vi "Zero.vi"(0 "PM NI568X in":refnum<class "Power Meter.lvclass">, 11 "error in (no error)":errorcluster) -> (4 "PM NI568X out":refnum<class "Power Meter.lvclass">, 15 "error out":errorcluster)   [LabVIEW 2023, in "NI-568x RF Power Meter.lvlib" / "Power Meter.lvclass"]
uses:
  Power Meter.lvclass
  Power Meter.lvclass/Power Meter.ctl
  Properties/Read Resource Name.vi
  <vilib>/Utility/error.llb/Error Cluster From Error Code.vi
  <vilib>/ErrorRing/Error Ring.xnode
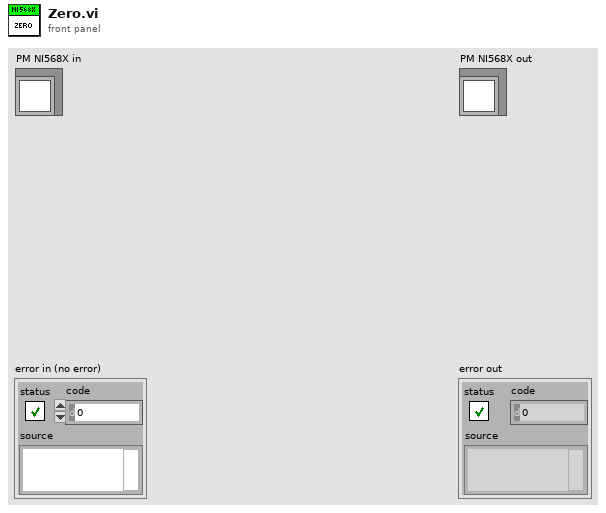
[diagram p1: front panel]
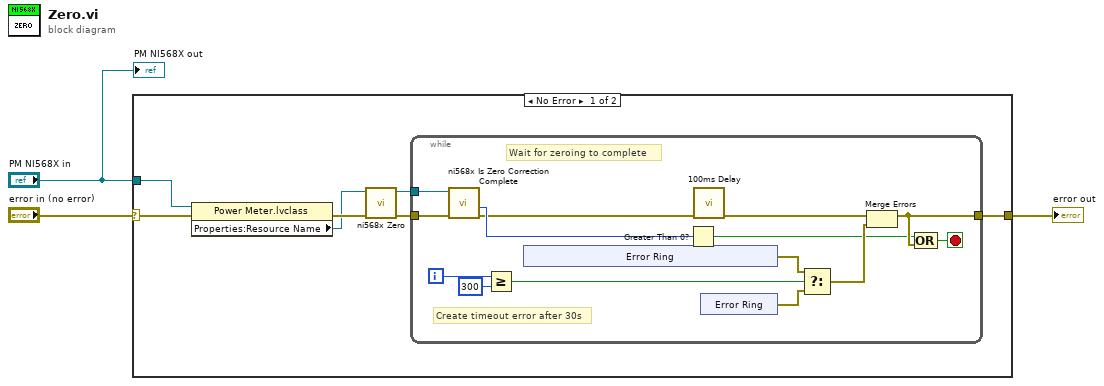
[diagram p0: block diagram]
diagram:
  n1 = case shown="No Error" "error in (no error)" {
    selector: "error in (no error)" -> [w7 w31]
    tunnel: [w8 w31] -> w3
    tunnel: "PM NI568X in" -> [w6 _]
    frame No Error {
      n2 = property class="Power Meter.lvclass"(reference=w6, error in=w7) -> (error out=w5:errorcluster, "Properties:Resource Name"=w4:refnum<k15>)  [unwired: 1 out]
      n3 = call <instrlib>:"ni568x Zero.vi"("error in"=w5, "instrument handle"=w4) -> ("error out"=w9:errorcluster, "instrument handle out"=w10:refnum<k15>)  [unwired: 8 in]
      n4 = while {
        tunnel: w9 -> [w24]
        tunnel: [w12] -> w8
        tunnel: w10 -> [w23]
        i -> [w22]
        stop <- w19 stop-if-true
        # "Create timeout error after 30s"
        # "Wait for zeroing to complete"
        n5 = call <instrlib>:"ni568x Is Zero Correction Complete.vi"("error in"=w24, "instrument handle"=w23) -> ("error out"=w18:errorcluster, "zero status"=w20:i32)  [unwired: 7 in, 1 out]
        n6 = Greater Or Equal?(x=w22, y=300) -> (x >= y?=w15:bool)
        n7 = xnode "Error Ring"() -> ("error out"=w16:errorcluster)
        n8 = Greater Than 0?(x=w20) -> (x > 0?=w11:bool)
        n9 = call "100ms Delay"("error in (no error)"=w18) -> ("error out"=w14:errorcluster)  [unwired: 10 in]
        n10 = xnode "Error Ring"() -> ("error out"=w17:errorcluster)
        n11 = Select(t=w16, s=w15, f=w17) -> (s? t:f=w13:errorcluster)
        n12 = Merge Errors(w14, w13) -> (w12:errorcluster)
        n13 = Compound Arithmetic op=OR(w11, w12) -> (w19:bool)
      }
    }
    frame Error {
    }
  }
  "error out" <- w3
  "PM NI568X out" <- "PM NI568X in"
